vi "integrate test2.vi"() -> ()   [LabVIEW 2020]
uses:
  <vilib>/Analysis/baseanly.llb/Mean (DBL).vi
  <vilib>/Analysis/NI_AALBase.lvlib
  <vilib>/measure/NI_MABase.lvlib
panel:
  in  "amplitude":dbl=1.0 format="%0.2p"
  in  "frequency":dbl=10.0 format="%0.2p"
  out "XY Graph 2":cluster{dbl[], "Amplitudes":dbl[]}[](graph)
  out "csapásszám":dbl format="%0.2f"
  out "original":waveform(dbl)(graph)
  out "impulse mean":dbl format="%0.2f"
  out "cutoff":waveform(dbl)(graph)
  out "XY Graph":cluster{"Ramp Pattern":dbl[], dbl[]}(graph)
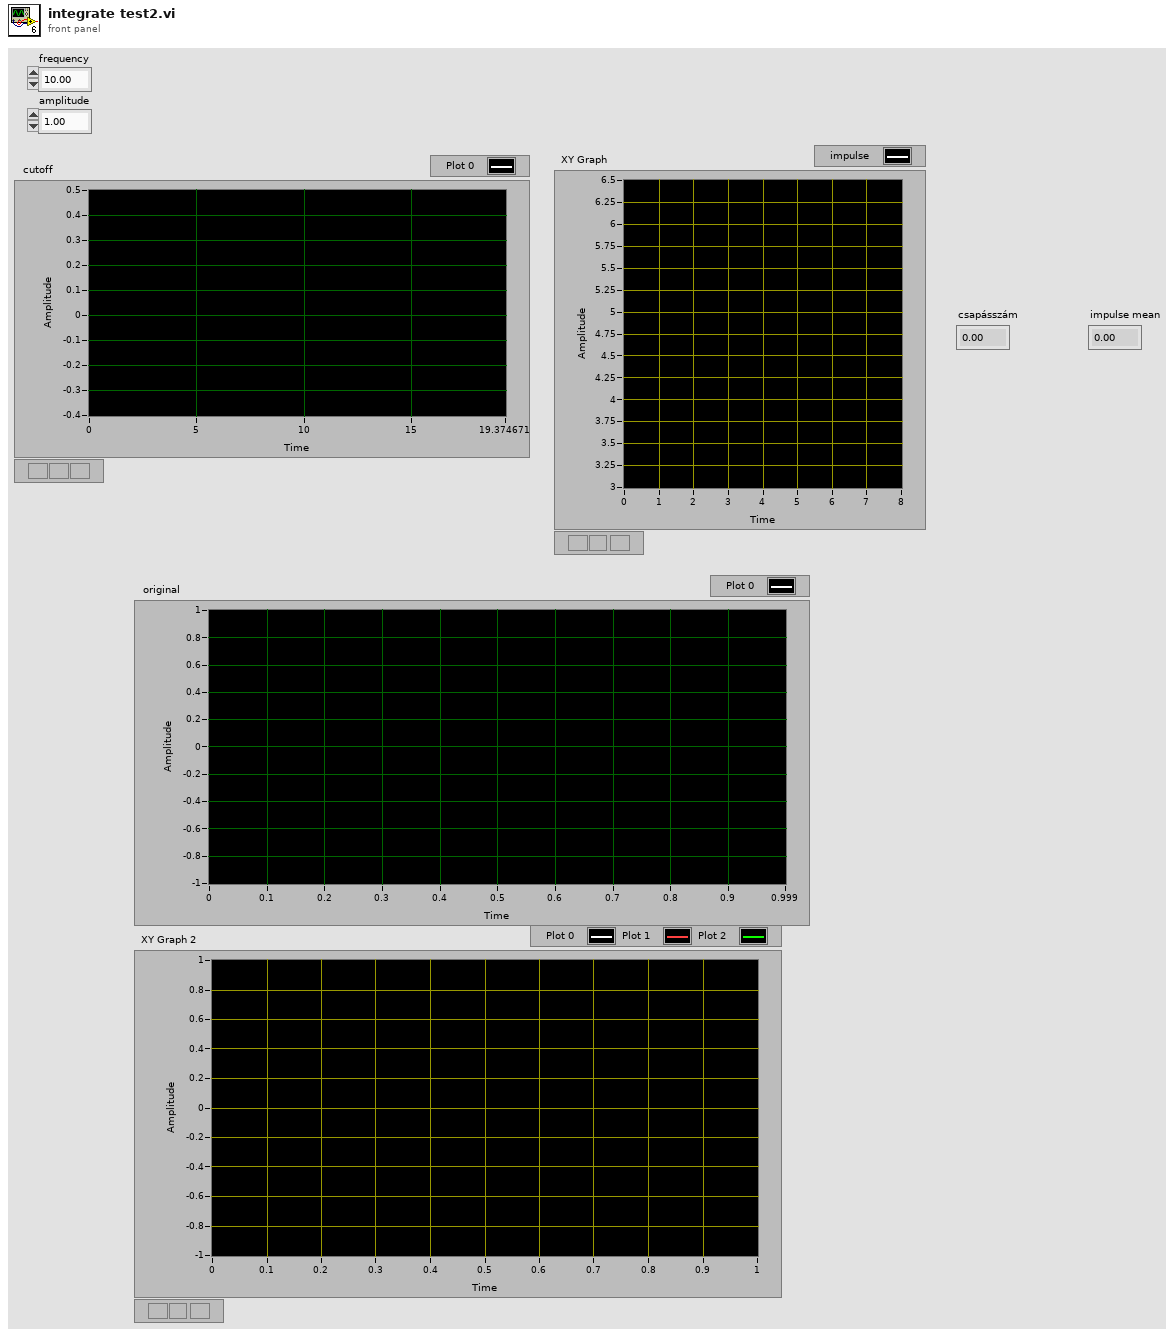
[diagram p1: front panel]
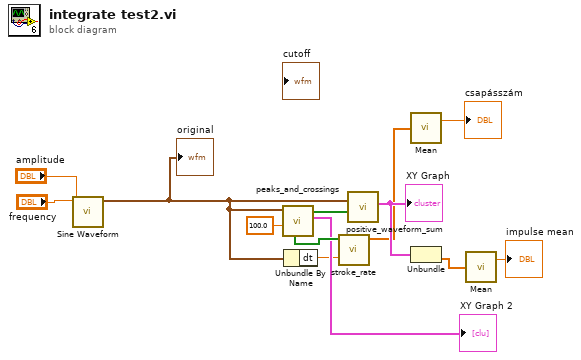
[diagram p0: block diagram]
diagram:
  n1 = call <vilib>:"Sine Waveform.vi"("amplitude"="amplitude", "frequency"="frequency") -> ("signal out"=w1:waveform(dbl))  [unwired: 8 in, 1 out]
  "original" <- w1
  n2 = call "peaks_and_crossings.vi"("end"=100.0, "waveform"=w1) -> ("all in array"=→"XY Graph 2":cluster{dbl[], "Amplitudes":dbl[]}[], "plus-minus crossing?"=w10:bool[], "minus-plus crossing?"=w9:bool[])  [unwired: 3 in, 4 out]
  n3 = Unbundle By Name(w1) -> ("dt"=w2:dbl)
  n4 = call "stroke_rate.vi"("dt"=w2, "minus-plus"=w9) -> ("stroke rate"=w8:dbl[])  [unwired: 9 in]
  n5 = call "positive_waveform_sum.vi"("plus-minus"=w10, "read in data"=w1) -> ("csapás impulzus"=w13:cluster{"Ramp Pattern":dbl[], dbl[]})  [unwired: 8 in, 1 out]
  "XY Graph" <- w13
  n6 = call-poly <vilib>:"Mean.vi"("X"=w8) -> ("mean"=→"csapásszám":dbl)  [unwired: 1 out]
  n7 = Unbundle(w13) -> (w12:dbl[])  [unwired: 1 out]
  n8 = call-poly <vilib>:"Mean.vi"("X"=w12) -> ("mean"=→"impulse mean":dbl)  [unwired: 1 out]
